vi "Practica6_Array.vi"() -> ()   [LabVIEW 2022 SP3]
panel:
  out "Indica lo del selector":cluster{"Valor5":dbl}
  out "array of clusters":cluster{"Valor5":dbl}[](array[cluster])
  out "Elementos del areglo":dbl(knob) scale=0.0..10.0
  in  "Valor5":dbl
  in  "Valor4":dbl
  in  "Valor3":dbl
  in  "Valor2":dbl
  in  "Valor1":dbl
  in  "Selector del dato":dbl
  # "Anahí Montserrat Vázquez Padilla \nPráctica 06: Array\n13/02/2024"
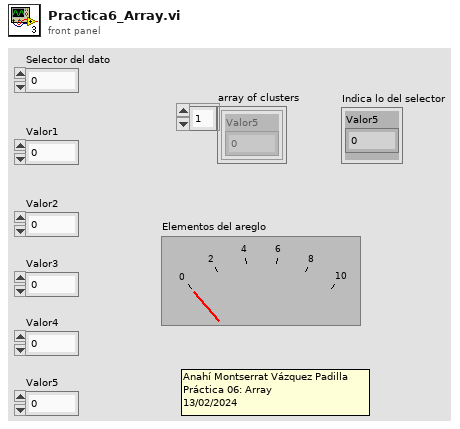
[diagram p1: front panel]
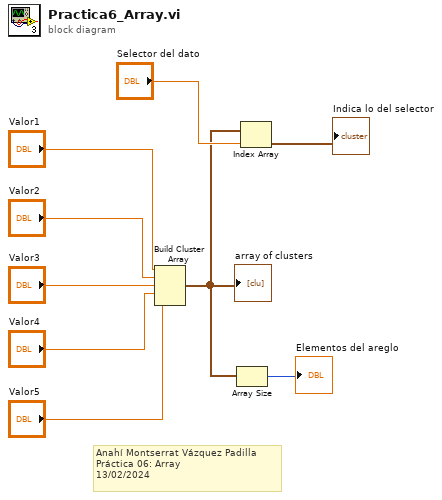
[diagram p0: block diagram]
diagram:
  # "Anahí Montserrat Vázquez Padilla \nPráctica 06: Array\n13/02/2024"
  n1 = Build Cluster Array("Valor1", "Valor2", "Valor3", "Valor4", "Valor5") -> (w3:cluster{"Valor5":dbl}[])
  "array of clusters" <- w3
  n2 = Array Size(array=w3) -> (size(s)=→"Elementos del areglo":i32)
  n3 = Index Array "Index Array"(array=w3, index="Selector del dato") -> (element=→"Indica lo del selector":cluster{"Valor5":dbl})
